vi "RunOperation.vi"(10 "Inputs":string[](array[string]), 11 "Test in":refnum<class "Test.lvclass">) -> (1 "Output/Failure":string, 2 "CLI Process Return Code":i32, 3 "Test out":refnum<class "Test.lvclass">)   [LabVIEW 2017, in "Test.lvclass"]
uses:
  Test.lvclass
  <vilib>/PNR/LVUnit/LVUnit Test Discoverer/LVUnit Test Discoverer.lvclass
  <vilib>/PNR/LVUnit/LVUnit Test Executor/LVUnit Test Executor.lvclass
  C:/Program Files (x86)/National Instruments/LabVIEW 2017/vi.lib/PNR/LVUnit/Test Executor/Test Executor.lvclass
  Test.lvclass/Test.ctl
  <vilib>/PNR/LVUnit/Test Executor/Test Executor.lvclass
  <vilib>/PNR/LVUnit/CodeCoverage/CodeCoverage.lvclass
  <vilib>/PNR/LVUnit/Cobertura/Cobertura.lvlib
  <vilib>/PNR/LVUnit/JUnit/JUnit.lvlib
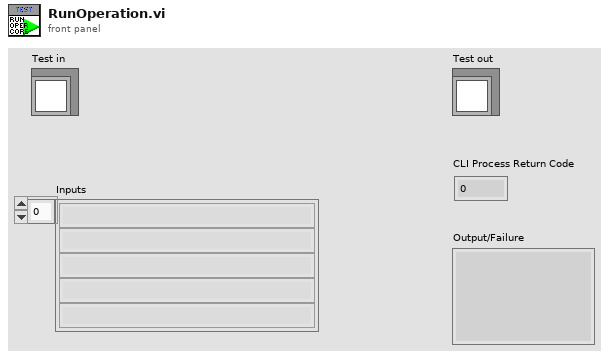
[diagram p1: front panel]
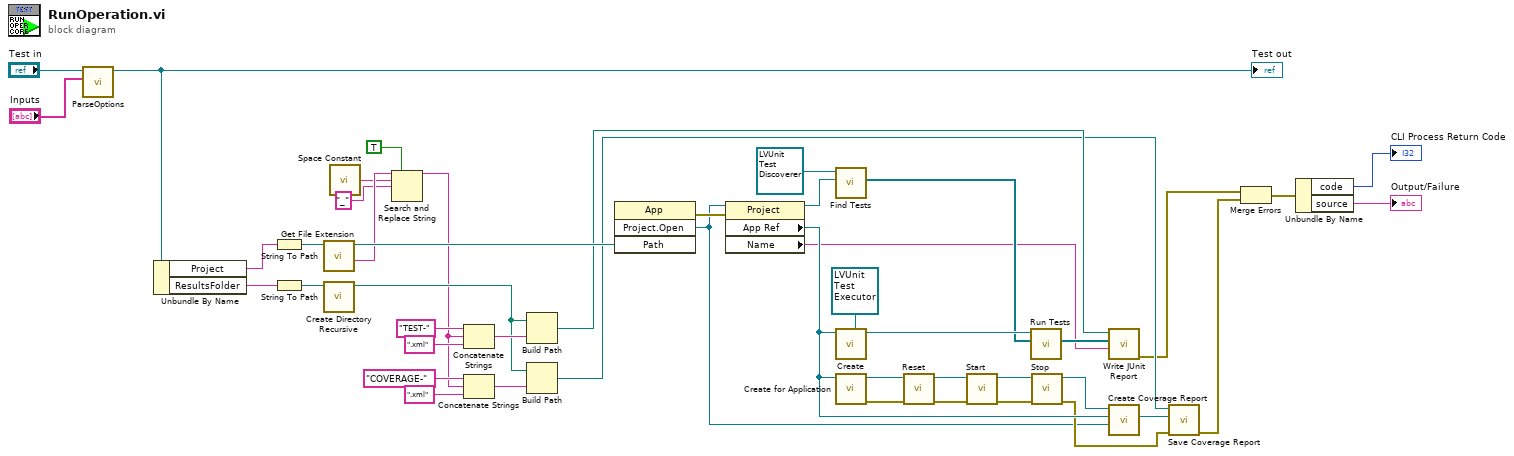
[diagram p0: block diagram]
diagram:
  n1 = call "ParseOptions.vi"("Options"="Inputs", "Test in"="Test in") -> ("Test out"=w42:refnum<class "Test.lvclass">)  [unwired: 8 in, 1 out]
  "Test out" <- w42
  n2 = Unbundle By Name(w42) -> ("Project"=w41:string, "ResultsFolder"=w39:string)
  n3 = String To Path(string=w41) -> (path=w37:path)
  n4 = String To Path(string=w39) -> (path=w38:path)
  n5 = call <vilib>:"Get File Extension.vi"("file"=w37) -> ("filename without extension"=w5:string, "dup file"=w33:path)  [unwired: 6 in, 3 out]
  n6 = call <vilib>:"Create Directory Recursive.vi"("directory"=w38) -> ("directory copy"=w17:path)  [unwired: 4 in, 2 out]
  n7 = call <vilib>:"Space Constant.vi"() -> ("String"=w4:string)
  n8 = Search and Replace String(replace all?=TRUE ("replace all? (F)"), input string=w5, search string=w4, replace string="_") -> (result string=w1:string)  [unwired: 4 in, 3 out]
  n9 = Concatenate Strings("TEST-" ("string"), w1, ".xml" ("string")) -> (w34:string)
  n10 = Concatenate Strings("COVERAGE-" ("string"), w1, ".xml" ("string")) -> (w18:string)
  n11 = Build Path(base path=w17, name or relative path=w34) -> (appended path=w21:path)
  n12 = Build Path(base path=w17, name or relative path=w18) -> (appended path=w15:path)
  n13 = invoke class="App" method="Project.Open"("Path"=w33) -> (error out=w40:errorcluster, "Project:Open"=w6:refnum<vi>)  [unwired: 3 in, 2 out]
  n14 = property class="Project"(reference=w6, error in=w40) -> (reference out=w30:refnum<vi>, "App Ref"=w23:refnum<vi>, "Name"=w7:string)  [unwired: 1 out]
  n15 = call-dynamic "Find Tests.vi"("Project Refnum"=w30, "LVUnit Test Discoverer in"=refnum<class "LVUnit Test Discoverer.lvclass"> refnum ("LVUnit Test Discoverer")) -> ("Test Cases"=w26:refnum<class "Test Case.lvclass">[])  [unwired: 7 in, 2 out]
  n16 = call <vilib>:"Create.vi"("Test Executor in"=refnum<class "LVUnit Test Executor.lvclass"> refnum ("LVUnit Test Executor"), "Application"=w23) -> ("Test Executor"=w27:refnum<class "LVUnit Test Executor.lvclass">)  [unwired: 8 in, 1 out]
  n17 = call <vilib>:"Create for Application.vi"("Application"=w23) -> ("error out"=w8:errorcluster, "CodeCoverage out"=w28:refnum<class "CodeCoverage.lvclass">)  [unwired: 9 in]
  n18 = call <vilib>:"Reset.vi"("error in (no error)"=w8, "CodeCoverage in"=w28) -> ("error out"=w9:errorcluster, "CodeCoverage out"=w29:refnum<class "CodeCoverage.lvclass">)  [unwired: 8 in]
  n19 = call <vilib>:"Start.vi"("error in (no error)"=w9, "CodeCoverage in"=w29) -> ("error out"=w10:errorcluster, "CodeCoverage out"=w25:refnum<class "CodeCoverage.lvclass">)  [unwired: 8 in]
  n20 = call-dynamic "Run Tests.vi"("Test Cases"=w26, "LVUnit Test Executor in"=w27) -> ("Test Results"=w22:refnum<class "Test Result.lvclass">[])  [unwired: 7 in, 2 out]
  n21 = call <vilib>:"Stop.vi"("error in (no error)"=w10, "CodeCoverage in"=w25) -> ("error out"=w11:errorcluster, "CodeCoverage out"=w24:refnum<class "CodeCoverage.lvclass">)  [unwired: 8 in]
  n22 = call <vilib>:"Write JUnit Report.vi"("Project Name"=w7, "Test Results"=w22, "File Path"=w21) -> ("error out"=w13:errorcluster)  [unwired: 8 in]
  n23 = call <vilib>:"Create Coverage Report.vi"("Project"=w6, "Application"=w23, "CodeCoverage in"=w24) -> ("Coverage"=w16:refnum<class "Coverage.lvclass">)  [unwired: 7 in, 1 out]
  n24 = call <vilib>:"Save Coverage Report.vi"("error in (no error)"=w11, "Coverage"=w16, "Path"=w15) -> ("error out"=w12:errorcluster)  [unwired: 8 in]
  n25 = Merge Errors(w13, w12) -> (w14:errorcluster)
  n26 = Unbundle By Name(w14) -> ("code"=→"CLI Process Return Code":i32, "source"=→"Output/Failure":string)
